vi "Midbrain Main.vi"(10 "QueueRef":T1, 11 "NotifierReff":T2) -> ()   [LabVIEW 2013]
uses:
  Data/TypeDefs/Notifiers.ctl
  Data/TypeDefs/UTM Location.ctl
  Data/TypeDefs/Sail Set Suggestions.ctl
  Data/TypeDefs/Rudder Set Suggestions.ctl
  Data/TypeDefs/OverrideInformation.ctl
  Data/TypeDefs/OverrideMode.ctl
  Data/TypeDefs/Queues.ctl
  Classes/Waypoint/Waypoint.lvclass
  Classes/Missions/GenericMission/GenericMission.lvclass
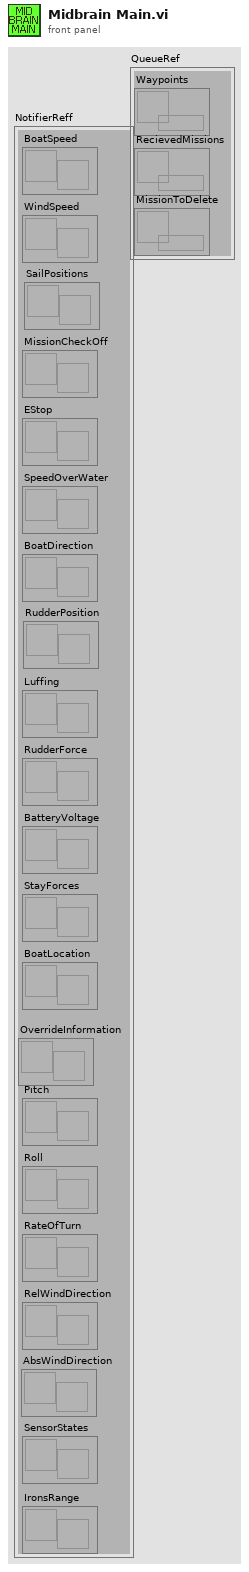
[diagram p1: front panel]
types:
  T1 = typedef "Queues.ctl" = cluster{"Waypoints":refnum<queue>, "RecievedMissions":refnum<queue>, "MissionToDelete":refnum<queue>}
  T2 = typedef "Notifiers.ctl" = cluster{"BoatSpeed":refnum<notifier>, "WindSpeed":refnum<notifier>, "MissionCheckOff":refnum<notifier>, "EStop":refnum<notifier>, "SpeedOverWater":refnum<notifier>, "BoatDirection":refnum<notifier>, "Luffing":refnum<notifier>, "RudderForce":refnum<notifier>, "BatteryVoltage":refnum<notifier>, "StayForces":refnum<notifier>, "BoatLocation":refnum<notifier>, "Pitch":refnum<notifier>, "Roll":refnum<notifier>, "RateOfTurn":refnum<notifier>, "RelWindDirection":refnum<notifier>, "SailPositions":refnum<notifier>, "RudderPosition":refnum<notifier>, "SensorStates":refnum<notifier>, "IronsRange":refnum<notifier>, "AbsWindDirection":refnum<notifier>, "OverrideInformation":refnum<notifier>}
  T3 = cluster{"AirmarOnline":bool, "WindvaneOnline":bool, "HemisphereOnline":bool, "RudderForceOnline":bool, "StayForceOnline":bool, "BatteryVoltageOnline":bool, "AccelerometerOnline":bool}
  T4 = typedef "Boat Regimes.ctl" = cluster{"Sailing Regime":T5, "Emergency Regimes":T6, "Emergency?":bool}
  T5 = typedef "Sailing Regimes.ctl" = enum16{"Tack - Bow across wind", "Upwind - Starboard Tack", "Turn between Upwind/Reach - Starboard Tack", "Reach - Starboard Tack", "Turn between Reach/Run - Starboard Tack", "Run - Starboard Tack", "Jibe - Stern across wind", "Run - Port Tack", "Turn between Reach/Run - Port Tack", "Reach - Port Tack", "Turn between Upwind/Reach - Port Tack", "Upwind - Port Tack"}
  T6 = typedef "Emergency Regimes.ctl" = enum16{"NO EMERGENCY", "No Knockdown", "Obstacle Avoid"}
  T7 = typedef "Rudder Set Suggestions.ctl" = dbl
  T8 = typedef "Sail Set Suggestions.ctl" = cluster{"MainSailSuggestion":dbl, "JibSailSuggestion":dbl}
  T9 = typedef "OverrideInformation.ctl" = cluster{"OverrideMode":T10, "SailSetting":T8, "Suggested Rudder Setpoint":T7}
  T10 = typedef "OverrideMode.ctl" = enum16{"None", "Rudder", "Sails", "Both"}
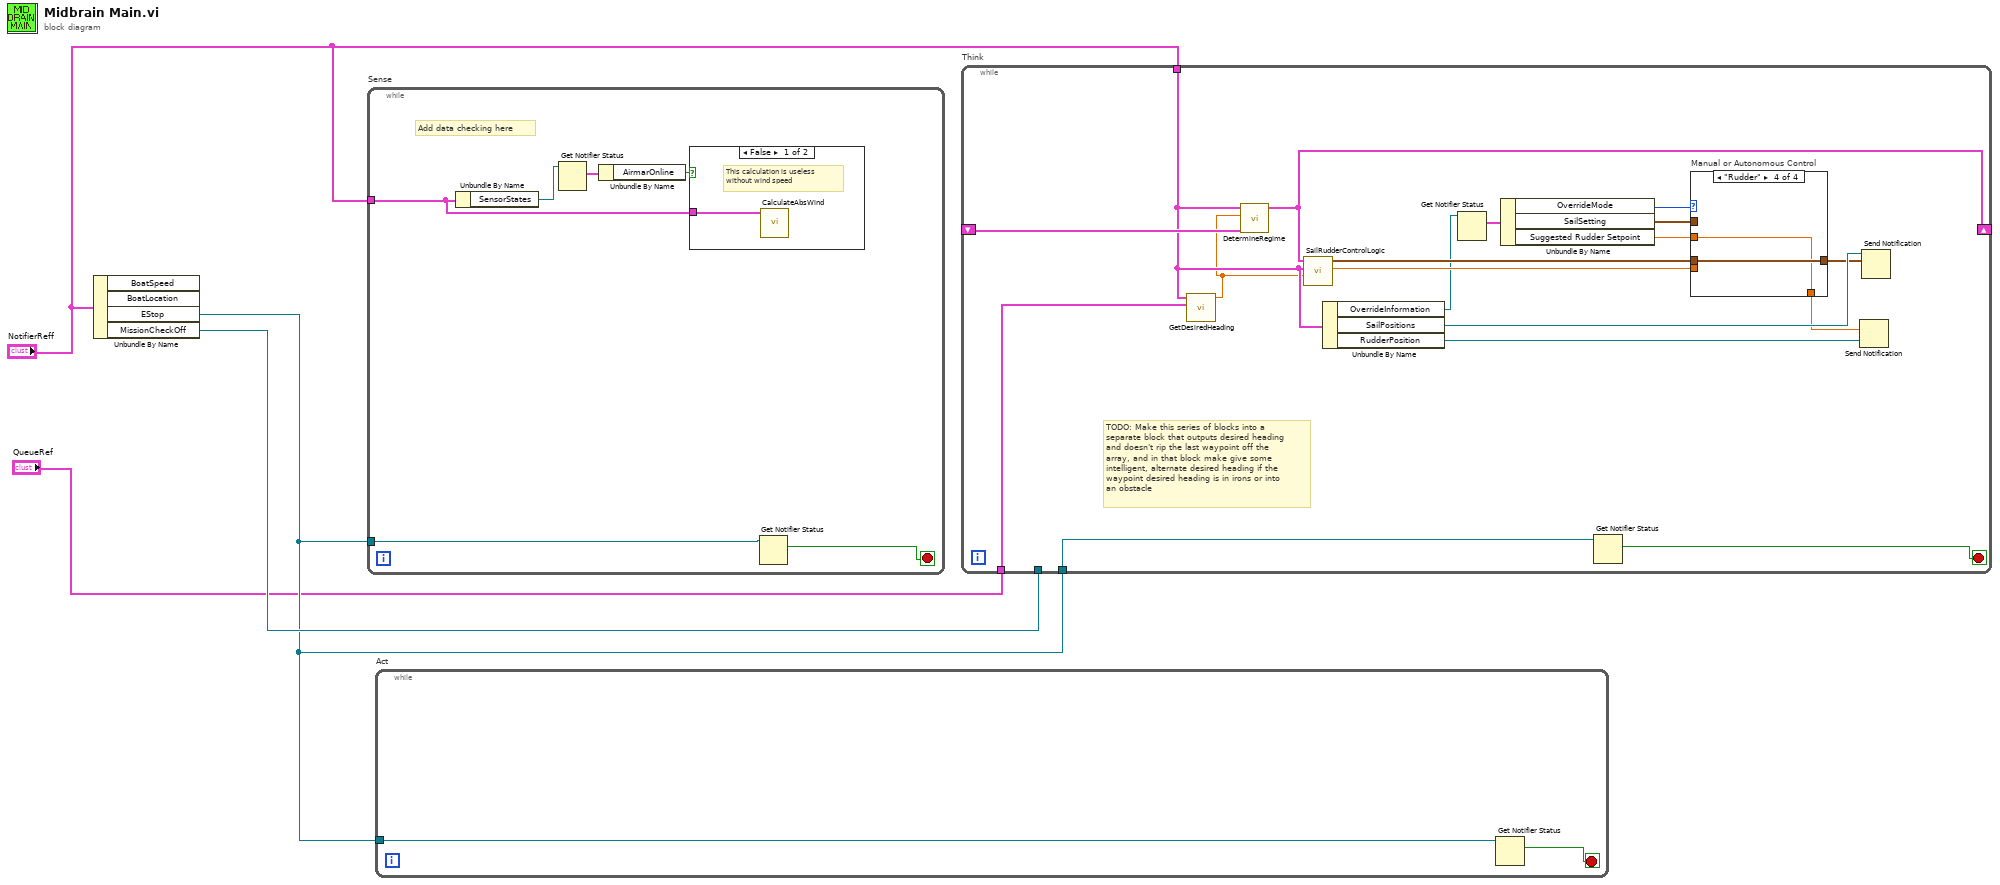
[diagram p0: block diagram]
diagram:
  n1 = Unbundle By Name("NotifierReff") -> ("EStop"=w3:refnum<notifier>, "MissionCheckOff"=w4:refnum<notifier>)  [unwired: 2 out]
  n2 = while "Sense" {
    tunnel: w3 -> [w10]
    tunnel: "NotifierReff" -> [w5]
    stop <- w9 stop-if-true
    # "Add data checking here"
    n3 = Unbundle By Name(w5) -> ("SensorStates"=w8:refnum<notifier>)
    n4 = Get Notifier Status(notifier=w8) -> (current notification=w7:T3)  [unwired: 1 in, 4 out]
    n5 = Unbundle By Name(w7) -> ("AirmarOnline"=w6:bool)
    n6 = case shown="False" w6 {
      tunnel: w5 -> [w11 _]
      frame False {
        # "This calculation is useless without wind speed"
        n7 = call "CalculateAbsWind.vi"("NotifierReff"=w11) -> ()  [unwired: 11 in]
      }
      frame True {
      }
    }
    n8 = Get Notifier Status(notifier=w10) -> (current notification=w9:bool)  [unwired: 1 in, 4 out]
  }
  n9 = while "Act" {
    tunnel: w3 -> [w13]
    stop <- w12 stop-if-true
    n10 = Get Notifier Status(notifier=w13) -> (current notification=w12:bool)  [unwired: 1 in, 4 out]
  }
  n11 = while "Think" {
    tunnel: w4 -> [_]
    tunnel: w3 -> [w31]
    shift-right: [w28] -> _
    shift-left: _ -> [w29]
    tunnel: "NotifierReff" -> [w25]
    tunnel: "QueueRef" -> [w23]
    stop <- w30 stop-if-true
    # "TODO: Make this series of blocks into a separate block that outputs desired heading and doesn't rip the last waypoint off the array, and in that block make give some intelligent, alternate desired heading if the waypoint desired heading is in irons or into an obstacle"
    n12 = call "GetDesiredHeading.vi"("QueueRef"=w23, "NotifierReff"=w25) -> ("Desired Heading"=w24:dbl)  [unwired: 9 in]
    n13 = call "DetermineRegime.vi"("Last Commanded Boat Regime"=w29, "Desired Heading (deg)"=w24, "NotifierReff"=w25) -> ("Commanded Boat Regime"=w28:T4)  [unwired: 8 in]
    n14 = call "SailRudderControlLogic.vi"("DesiredHeading"=w24, "NotifierReff"=w25, "Commanded Boat Regime"=w28) -> ("Suggested Rudder Setpoint"=w20:T7, "Suggested Sail Setpoints"=w22:T8)  [unwired: 7 in]
    n15 = Unbundle By Name(w25) -> ("OverrideInformation"=w18:refnum<notifier>, "SailPositions"=w26:refnum<notifier>, "RudderPosition"=w27:refnum<notifier>)
    n16 = Get Notifier Status(notifier=w18) -> (current notification=w17:T9)  [unwired: 1 in, 4 out]
    n17 = Unbundle By Name(w17) -> ("OverrideMode"=w16:T10, "SailSetting"=w15:T8, "Suggested Rudder Setpoint"=w14:T7)
    n18 = Get Notifier Status(notifier=w31) -> (current notification=w30:bool)  [unwired: 1 in, 4 out]
    n19 = case "Manual or Autonomous Control" shown="\"Rudder\"" w16 {
      tunnel: w22 -> [w33 _ _ w39]
      tunnel: [w33 w35 w37 w39] -> w21
      tunnel: w20 -> [w32 w34 _ _]
      tunnel: [w32 w34 w36 w38] -> w19
      tunnel: w15 -> [_ w35 w37 _]
      tunnel: w14 -> [_ _ w36 w38]
      frame "None", Default {
      }
      frame "Sails" {
      }
      frame "Both" {
      }
      frame "Rudder" {
      }
    }
    n20 = Send Notification(notification=w19, notifier=w27) -> ()  [unwired: 1 in, 2 out]
    n21 = Send Notification(notification=w21, notifier=w26) -> ()  [unwired: 1 in, 2 out]
  }
